vi "PovHelper.vi"(11 "Input POV":dbl) -> (0 "Left arrow":bool, 1 "Down arrow":bool, 2 "Right arrow":bool, 3 "Top arrow":bool)   [LabVIEW 2015]
panel:
  # "0 is the top arrow and it goes around \nclockwise"
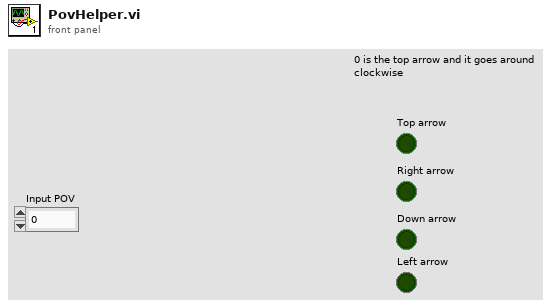
[diagram p1: front panel]
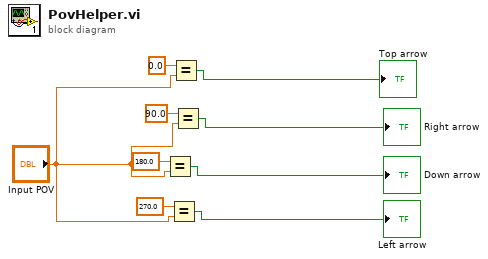
[diagram p0: block diagram]
diagram:
  n1 = Equal?(x=180.0, y="Input POV") -> (x = y?=→"Down arrow":bool)
  n2 = Equal?(x=270.0, y="Input POV") -> (x = y?=→"Left arrow":bool)
  n3 = Equal?(x=0.0, y="Input POV") -> (x = y?=→"Top arrow":bool)
  n4 = Equal?(x=90.0, y="Input POV") -> (x = y?=→"Right arrow":bool)
